vi "Split DAQ Data.vi"(0 "L1 Absolute Offsets":dbl[](array[numeric]), 1 "L1 Measured Sensitivities":dbl[](array[numeric]), 2 "Number of LBCBs":T1, 5 "Responses":dbl[](array[numeric]), 9 "L2 Absolute Offsets":dbl[](array[numeric]), 11 "L2 Measured Sensitivities":dbl[](array[numeric]), 12 "Number of \nExternal \nChannels":i32) -> (4 "Servo Error":dbl[][](array[numeric]), 6 "LVDT & LC":dbl[][](array[numeric]), 8 "External Channels":dbl[](array[numeric]), 10 "Volts LVDT & LC":dbl[][](array[numeric]), 15 "External Actuator Channels":dbl[](array[numeric]))   [LabVIEW 2009]
uses:
  Data Access Objects/Application/Number Of LBCBs.ctl
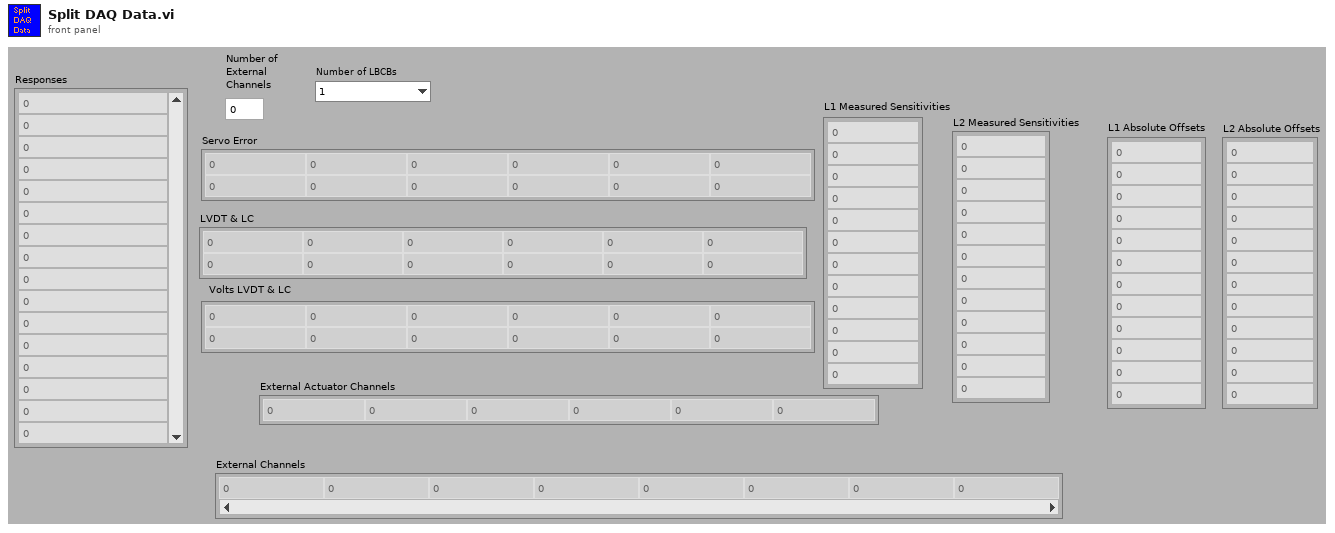
[diagram p1: front panel]
types:
  T1 = typedef "Number Of LBCBs.ctl" = enum16{"1", "2"}
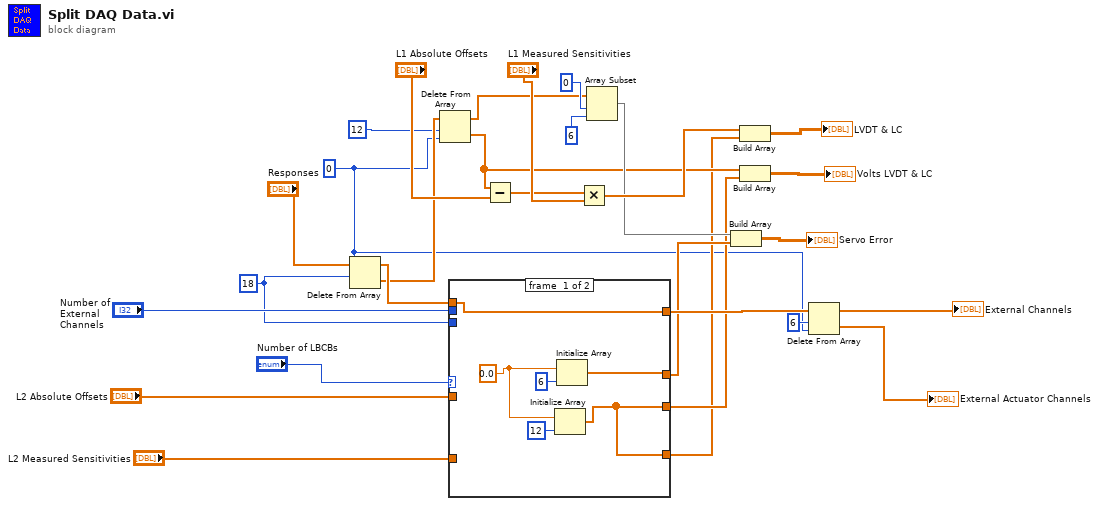
[diagram p0: block diagram]
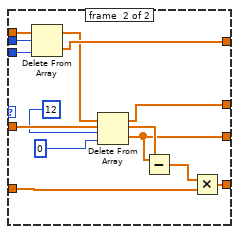
[diagram p2: hidden frame]
diagram:
  w2 = 0 ("index")
  w20 = 18
  n1 = Delete From Array(array="Responses", length=w20, index=w2) -> (deleted portion=w16:dbl[], array with subset deleted=w19:dbl[])
  n2 = Delete From Array(array=w16, length=12, index=w2) -> (deleted portion=w15:dbl[], array with subset deleted=w14:dbl[])
  n3 = case shown="\"2\"" "Number of LBCBs" {
    tunnel: [w31 w48] -> w5
    tunnel: [w30 w47] -> w9
    tunnel: [w35 w46] -> w28
    tunnel: "L2 Absolute Offsets" -> [_ w45]
    tunnel: "L2 Measured Sensitivities" -> [_ w44]
    tunnel: [w31 w39] -> w7
    tunnel: "Number of \nExternal \nChannels" -> [_ w38]
    tunnel: w20 -> [_ w37]
    tunnel: w19 -> [w35 w36]
    frame #0 {
      w34 = 0.0
      n4 = Initialize Array(w34, 12 ("dimension size")) -> (w31:dbl[])
      n5 = Initialize Array(w34, 6 ("dimension size")) -> (w30:dbl[])
    }
    frame #1 {
      n6 = Delete From Array(array=w36, length=w38, index=w37) -> (deleted portion=w46:dbl[], array with subset deleted=w43:dbl[])
      n7 = Delete From Array(array=w43, length=12, index=0) -> (deleted portion=w39:dbl[], array with subset deleted=w47:dbl[])
      n8 = Subtract(x=w39, y=w45) -> (x-y=w42:dbl[])
      n9 = Multiply(x=w42, y=w44) -> (x*y=w48:dbl[])
    }
  }
  n10 = Subtract(x=w15, y="L1 Absolute Offsets") -> (x-y=w12:dbl[])
  n11 = Multiply(x=w12, y="L1 Measured Sensitivities") -> (x*y=w27:dbl[])
  n12 = Array Subset(array=w14, index=0, length=6) -> (w26:dbl[])
  n13 = Build Array(w26, w9) -> (→"Servo Error":dbl[][])
  n14 = Build Array(w27, w5) -> (→"LVDT & LC":dbl[][])
  n15 = Build Array(w15, w7) -> (→"Volts LVDT & LC":dbl[][])
  n16 = Delete From Array(array=w28, length=6, index=w2) -> (deleted portion=→"External Actuator Channels":dbl[], array with subset deleted=→"External Channels":dbl[])
